vi "libssh2_channel_free.vi"(8 "error in (no error)":errorcluster, 11 "channel":T1) -> (0 "error out":errorcluster, 3 "return value":i32)   [LabVIEW 2013, in "libssh2.lvlib"]
doc: "Frees all resouces associated with a channel."
uses:
  libssh2.lvlib
  Channel Refnum.ctl
  libssh2.dll
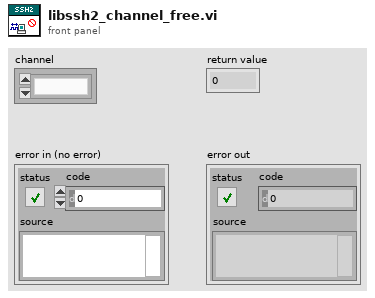
[diagram p1: front panel]
types:
  T1 = typedef "libssh2.lvlib/Channel Refnum.ctl" = refnum<k1>
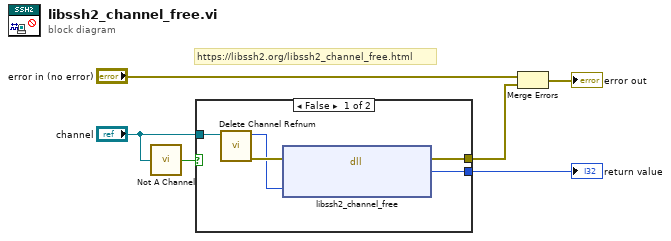
[diagram p0: block diagram]
diagram:
  # "https://libssh2.org/libssh2_channel_free.html"
  n1 = call "Not A Channel.vi"("channel"="channel") -> ("Not a Channel?"=w1:bool)
  n2 = case shown="False" w1 {
    tunnel: [w11 _] -> w6
    tunnel: "channel" -> [w8 _]
    tunnel: [w7 _] -> w5
    frame False {
      n3 = call "Delete Channel Refnum.vi"("channel"=w8) -> ("error out"=w10:errorcluster, "LIBSSH2_CHANNEL*"=w9:u64)  [unwired: 9 in]
      n4 = dll-call lib="C:/Users/pasca/source/repos/libssh2-labview/libssh2**.*" fn="libssh2_channel_free"(error in=w10, "channel"=w9) -> (error out=w7:errorcluster, "return value"=w11:i32)  [unwired: 3 in, 1 out]
    }
    frame True {
    }
  }
  "return value" <- w6
  n5 = Merge Errors("error in (no error)", w5) -> (→"error out":errorcluster)
